vi "GetBufferCapacity.vi"(7 "SMU":T1, 8 "Error In":errorcluster, 10 "Buffer":u8=1 min=1 max=2 step=1, 11 "Kiethley 2602 In":refnum<visa-resource-name>) -> (0 "Error Out":errorcluster, 2 "Number of Readings":i32, 3 "Keithley 2602 Out":refnum<visa-resource-name>)   [LabVIEW 2012, in "Keithley-2602.lvlib"]
uses:
  Keithley-2602.lvlib
  Controls/SMU.ctl
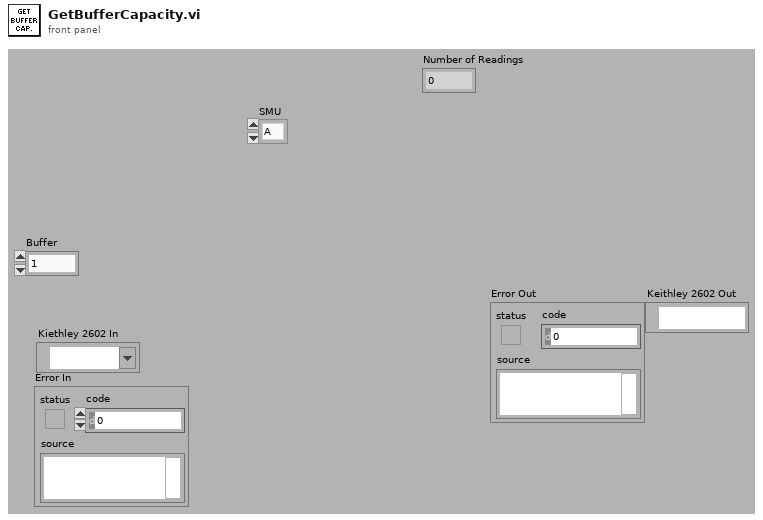
[diagram p1: front panel]
types:
  T1 = typedef "Keithley-2602.lvlib/SMU.ctl" = enum16{"A", "B"}
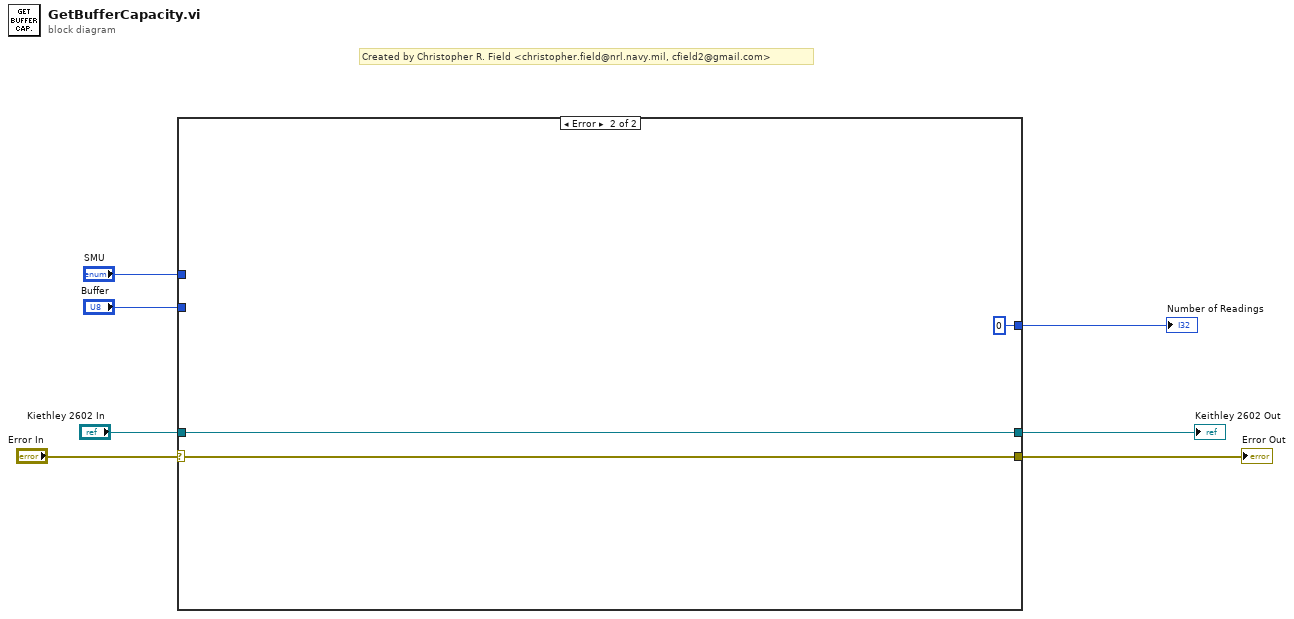
[diagram p0: block diagram]
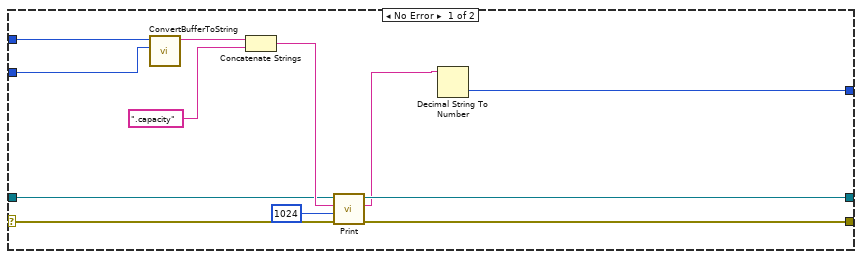
[diagram p2: hidden frame]
diagram:
  # "Created by Christopher R. Field <christopher.field@nrl.navy.mil, cfield2@gmail.com>"
  n1 = case shown="Error" "Error In" {
    selector: "Error In" -> [w9 w22]
    tunnel: "Kiethley 2602 In" -> [w17 w21]
    tunnel: [w16 w21] -> w6
    tunnel: "Buffer" -> [w15 _]
    tunnel: [w11 0] -> w4
    tunnel: "SMU" -> [w10 _]
    tunnel: [w8 w22] -> w1
    frame No Error {
      n2 = call "ConvertBufferToString.vi"("Buffer"=w15, "SMU"=w10) -> ("Buffer"=w14:string)  [unwired: 9 in]
      n3 = Concatenate Strings(w14, ".capacity" ("string")) -> (w19:string)
      n4 = call "Print.vi"("Error In"=w9, "Byte Count"=u32 1024, "Attribute"=w19, "Kiethley 2602 In"=w17) -> ("Error Out"=w8:errorcluster, "Output"=w12:string, "Keithley 2602 Out"=w16:refnum<visa-resource-name>)  [unwired: 5 in]
      n5 = Decimal String To Number(string=w12) -> (number=w11:i32)  [unwired: 2 in, 1 out]
    }
    frame Error {
    }
  }
  "Keithley 2602 Out" <- w6
  "Number of Readings" <- w4
  "Error Out" <- w1
